vi "led_off.vi"(8 "CurrentState":string, 11 "Action":enum16{"Entry", "During", "Exit"}(ring)) -> (0 "NextState":string)   [LabVIEW 2021]
uses:
  led_globals.vi
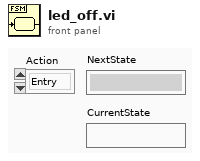
[diagram p1: front panel]
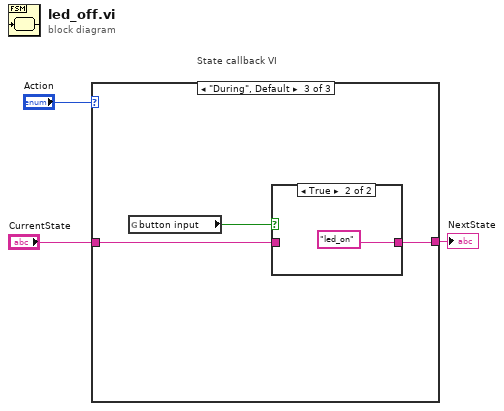
[diagram p0: block diagram]
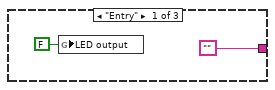
[diagram p2: hidden frame]
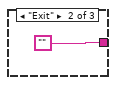
[diagram p3: hidden frame]
diagram:
  # "State callback VI"
  n1 = case shown="\"During\", Default" "Action" {
    tunnel: ["" "" w8] -> w2
    tunnel: "CurrentState" -> [_ _ w7]
    frame "Entry" {
      n2 = global write "led_globals.vi" "LED output"(FALSE ("LED output")) -> ()
    }
    frame "Exit" {
    }
    frame "During", Default {
      n3 = global read "led_globals.vi" "button input"() -> (w9:bool)
      n4 = case shown="True" w9 {
        tunnel: [w10 "led_on"] -> w8
        tunnel: w7 -> [w10 _]
        frame False {
        }
        frame True {
        }
      }
    }
  }
  "NextState" <- w2
